vi "Nernst T to R.vi"(10 "Temperature (C)":dbl format="%#_13g") -> (2 "Resistance (Ohms)":dbl)   [LabVIEW 2014, in "UEGO Sim Engine.lvlib"]
uses:
  UEGO Sim Engine.lvlib
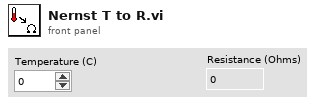
[diagram p1: front panel]
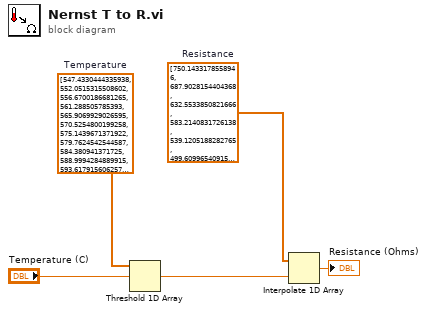
[diagram p0: block diagram]
diagram:
  w5 = dbl[] [750.1433178558946, 687.9028154404368, 632.5533850821666, 583.2140831726138, 539.1205188282765, 499.6099654091522, 464.1082722716965, 432.1183674503118, 403.21016610087827, 377.0117206661962, 353.2014676972758, 331.5014427213464, 311.6713493888965, 293.5033820194658, 276.81771234888583, 261.4585613507079, 247.29078609822318, 234.19691970164422, 222.07460936787538, 210.8344040052034, 200.39784832834266, 190.69584543642122, 181.66725414025132, 173.25769132224377, 165.4185130050173, 158.10595084226225, 151.2803836251842, 144.90572555409744, 138.94891549320891, 133.37949300429318, 128.16924890317023, 123.29193942307029, 118.72305444674566, 114.43963146582246, 110.42010792158544, 106.64420556812547, 103.09284123213729, 99.74805912608281, 96.59298053820385, 93.6117672000546, 90.78959519258933, 88.11263669608161, 85.56804726243718, 83.14395660004811, 80.8294612224563, 78.61461755243363, 76.49043427308789, 74.44886297220364, 72.48278625280363, 70.58600271661999, 68.75320824532537, 66.97997323068557, 65.26271545398049, 63.598668405087665, 61.98584492178634, 60.42299606354209, 58.90956525760703, 57.445637693221215, 56.64722373287076, 55.84880977252033, 55.05039581216988, 54.25198185181943, 53.453567891469, 52.65515393111855, 51.856739970768096, 51.058326010417666, 50.259912050067214, 49.46149808971676, 48.663084129366325, 47.864670169015895, 47.06625620866542, 46.26784224831499, 45.46942828796456, 44.67101432761409, 43.87260036726366, 43.07418640691323, 42.275772446562755, 41.477358486212324, 41.13613608826854, 40.79491369032476, 40.453691292380974, 40.11246889443719, 39.771246496493404, 39.43002409854962, 39.08880170060584, 38.747579302662054, 38.406356904718265, 38.06513450677449, 37.7239121088307, 37.382689710886915, 37.04146731294313, 36.700244914999345, 36.359022517055564, 36.01780011911178, 35.676577721167995, 35.335355323224206, 34.99413292528043, 34.652910527336644, 34.31168812939205, 33.97046573144827]  # Resistance
  w3 = dbl[] [547.4330444335938, 552.0515315508602, 556.6700186681265, 561.288505785393, 565.9069929026595, 570.5254800199258, 575.1439671371922, 579.7624542544587, 584.380941371725, 588.9994284889915, 593.6179156062578, 598.2364027235243, 602.8548898407907, 607.4733769580571, 612.0918640753235, 616.71035119259, 621.3288383098563, 625.9473254271228, 630.5658125443892, 635.1842996616556, 639.802786778922, 644.4212738961885, 649.0397610134548, 653.6582481307213, 658.2767352479877, 662.8952223652541, 667.5137094825205, 672.132196599787, 676.7506837170533, 681.3691708343198, 685.9876579515862, 690.6061450688526, 695.224632186119, 699.8431193033855, 704.4616064206518, 709.0800935379183, 713.6985806551846, 718.3170677724511, 722.9355548897175, 727.5540420069839, 732.1725291242503, 736.7910162415167, 741.4095033587831, 746.0279904760496, 750.6464775933159, 755.2649647105824, 759.8834518278488, 764.5019389451152, 769.1204260623816, 773.7389131796481, 778.3574002969144, 782.9758874141809, 787.5943745314473, 792.2128616487137, 796.8313487659801, 801.4498358832466, 806.0683230005129, 810.6868101177794, 815.3052972350458, 819.9237843523122, 824.5422714695786, 829.1607585868451, 833.7792457041114, 838.3977328213779, 843.0162199386443, 847.6347070559107, 852.2531941731771, 856.8716812904436, 861.4901684077099, 866.1086555249763, 870.7271426422428, 875.3456297595092, 879.9641168767755, 884.5826039940421, 889.2010911113084, 893.8195782285748, 898.4380653458413, 903.0565524631077, 907.675039580374, 912.2935266976405, 916.9120138149069, 921.5305009321733, 926.1489880494397, 930.7674751667062, 935.3859622839725, 940.004449401239, 944.6229365185054, 949.2414236357718, 953.8599107530382, 958.4783978703047, 963.096884987571, 967.7153721048375, 972.3338592221039, 976.9523463393703, 981.5708334566367, 986.1893205739032, 990.8078076911695, 995.426294808436, 1000.0447819257024, 1004.6632690429688]  # Temperature
  n1 = Threshold 1D Array(2:"Temperature (C)", 3:w3) -> (0:w4:dbl)  [unwired: 1 in]
  n2 = Interpolate 1D Array(1:w4, 2:w5) -> (0:→"Resistance (Ohms)":dbl)
